vi "Init DAQ PWM.vi"(8 "error in":errorcluster, 11 "physical channels":tag="Dev2/ai0") -> (0 "error out":errorcluster, 3 "Refnum out":refnum<k21>)   [LabVIEW 2021]
uses:
  <vilib>/DAQmx/create/channels.llb/DAQmx Create Channel (CO-Pulse Generation-Frequency).vi
panel:
  in  "duty cycle":dbl=0.5 format="%.6f"
  in  "frequency":dbl=1.0 format="%.6f"
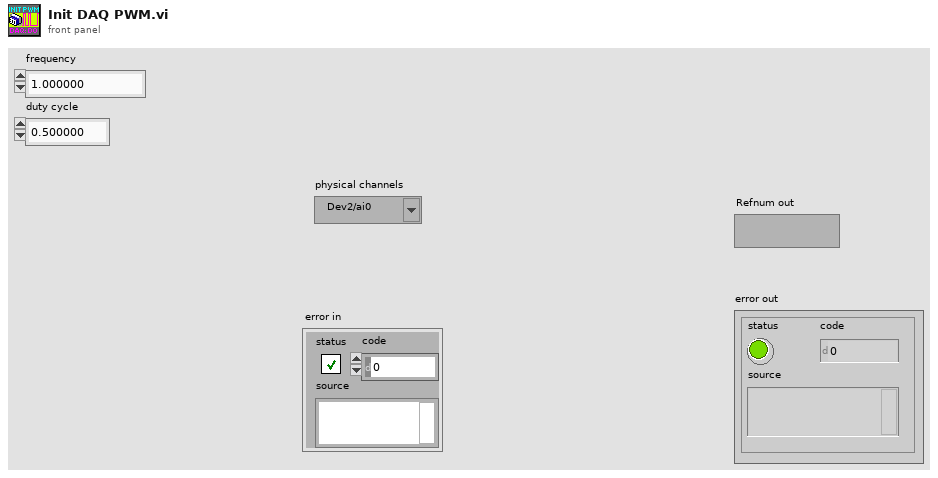
[diagram p1: front panel]
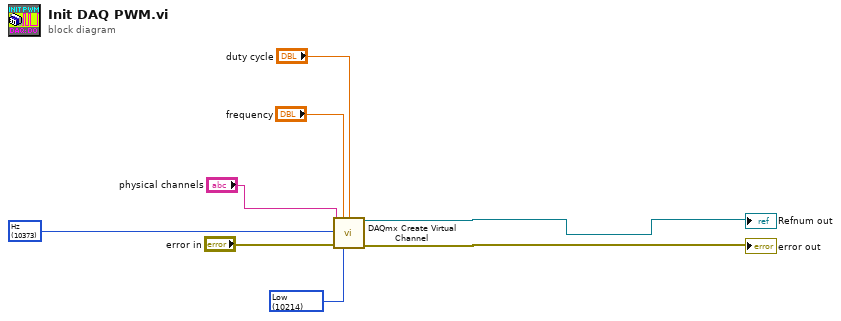
[diagram p0: block diagram]
diagram:
  w1 = 10214 items=["High"=10192, "Low"=10214] ("idle state")
  w2 = 10373 items=["Hz"=10373] ("units")
  n1 = call-poly <vilib>:"DAQmx Create Virtual Channel.vi"("frequency"="frequency", "duty cycle"="duty cycle", "counter"="physical channels", "units"=w2, "error in"="error in", "idle state"=w1) -> ("task out"=→"Refnum out":refnum<k21>, "error out"=→"error out":errorcluster)  [unwired: 8 in]
